vi "Parcial_Elevador.vi"() -> ()   [LabVIEW 2024]
uses:
  <vilib>/Utility/miscctls.llb/LVPositionTypeDef.ctl
panel:
  out "Position 2":T1
  in  "Position":T1={"Left"=400, "Top"=470}
  in  "Stop Button":bool
  in  "2 Piso Button":bool
  in  "3 Piso Button":bool
  in  "1 Piso Button":bool
  out "Elevador":bool
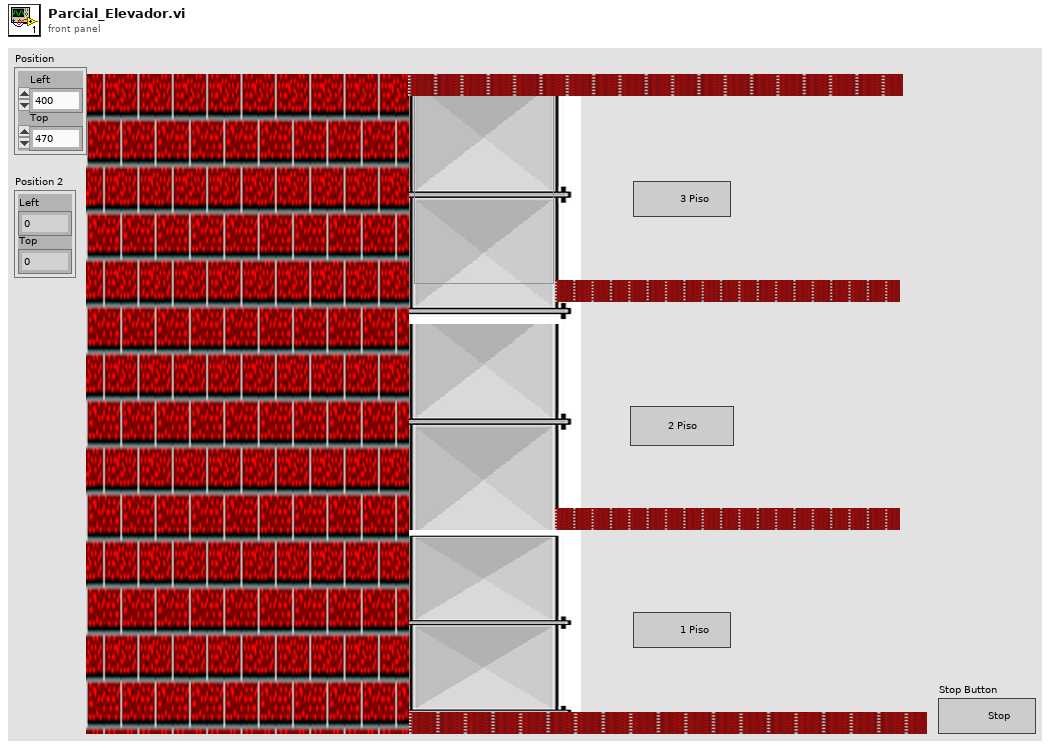
[diagram p1: front panel]
types:
  T1 = typedef "LVPositionTypeDef.ctl" = cluster{"Left":i32, "Top":i32}
  T2 = enum16{"Inicio", "1", "2 Subiendo", "3", "2 Bajando"}
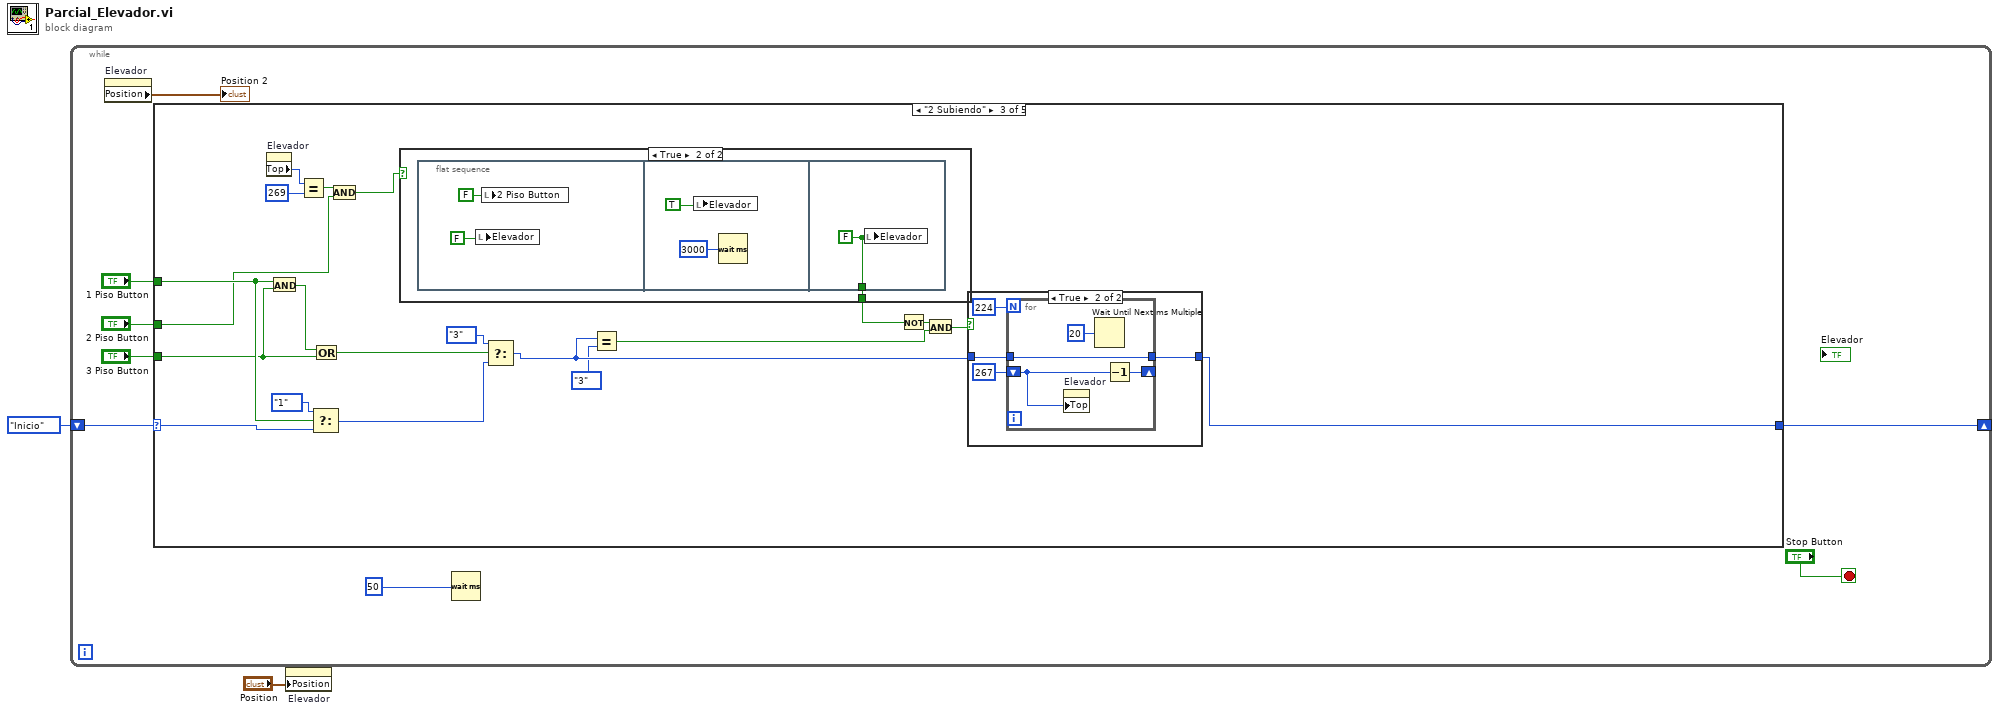
[diagram p0: block diagram]
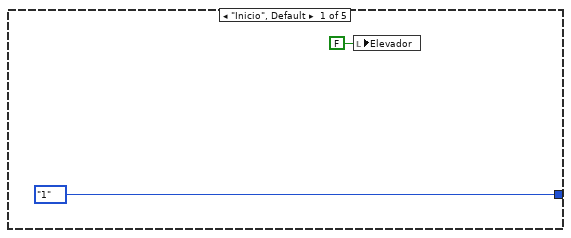
[diagram p2: hidden frame]
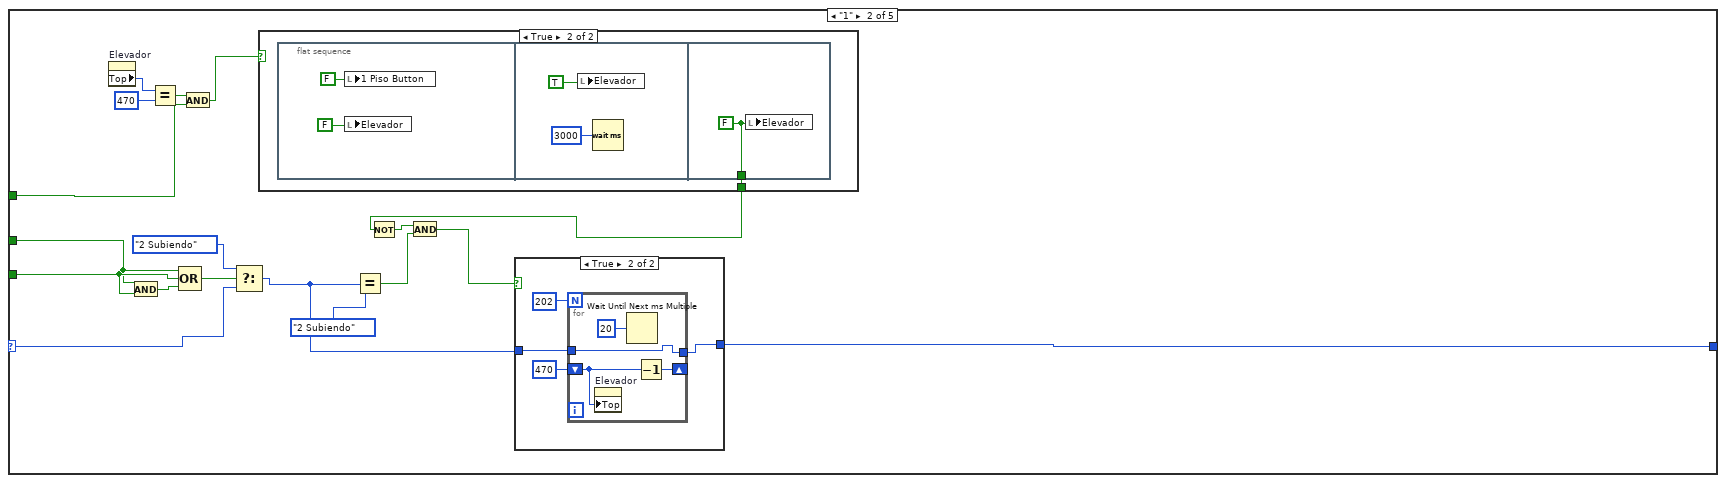
[diagram p3: hidden frame]
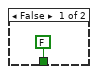
[diagram p5: hidden frame]
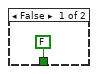
[diagram p6: hidden frame]
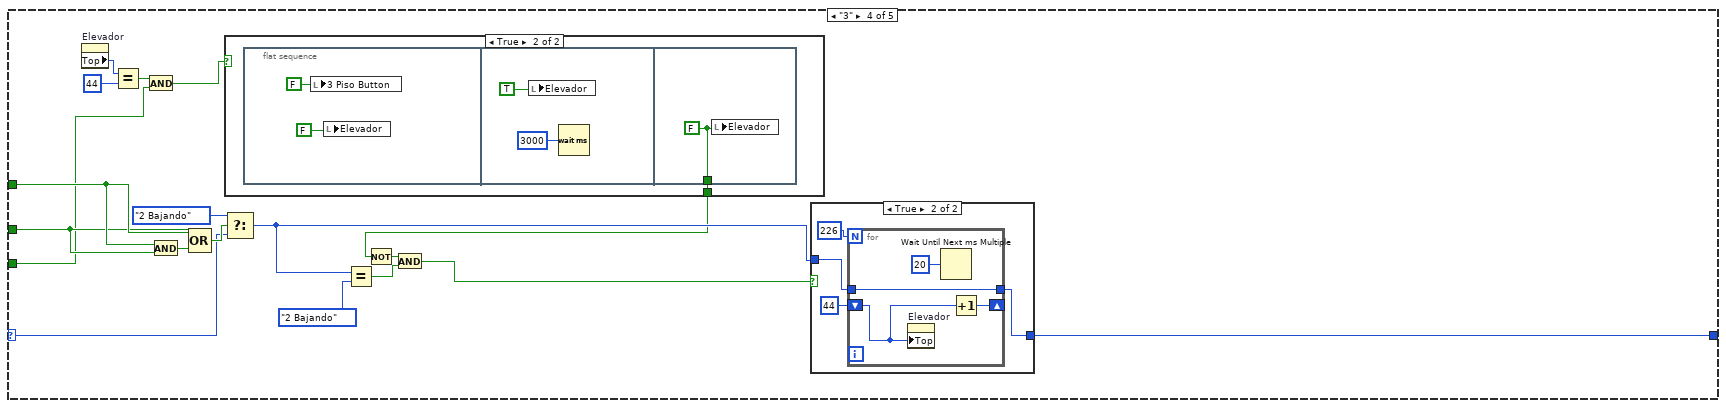
[diagram p8: hidden frame]
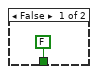
[diagram p9: hidden frame]
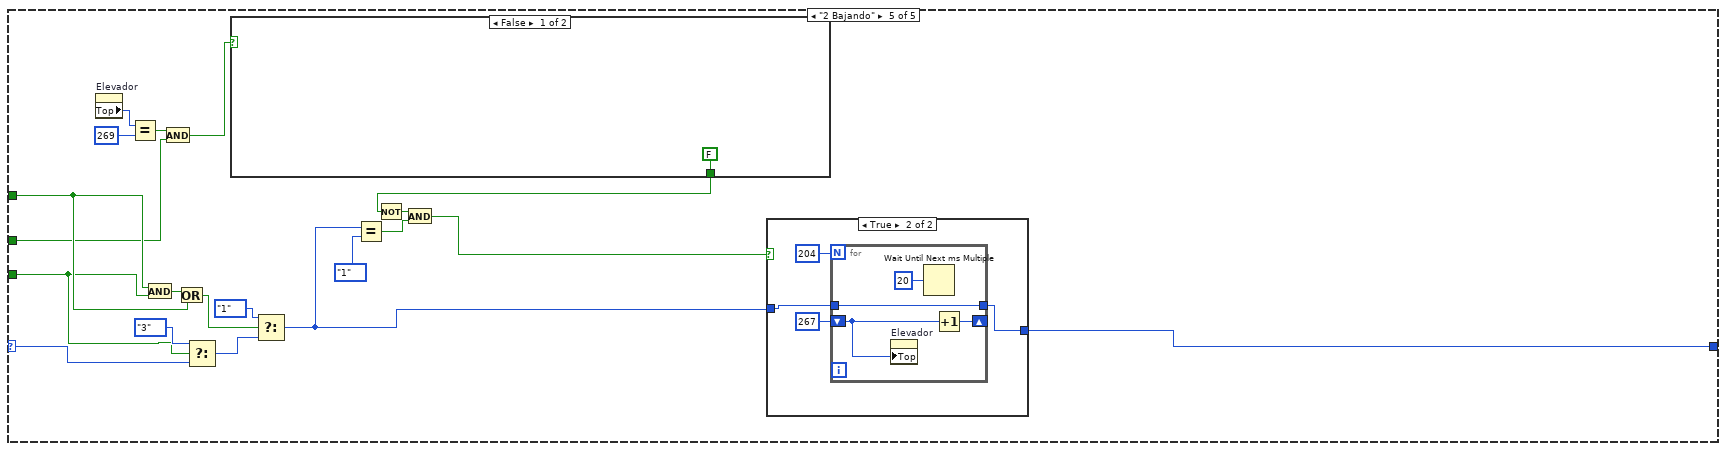
[diagram p11: hidden frame]
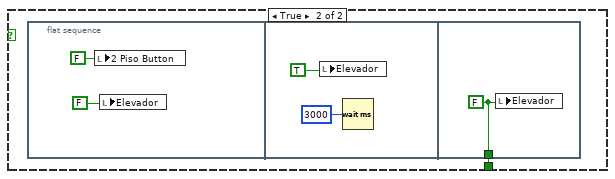
[diagram p12: hidden frame]
diagram:
  n1 = while {
    shift-right: [w4] -> _
    shift-left: T2."Inicio" -> [w9]
    stop <- "Stop Button" stop-if-true
    n2 = property on="Elevador" class="Bool (strict)"() -> ("Position"=→"Position 2":T1)  [unwired: 2 in, 2 out]
    n3 = case shown="\"2 Subiendo\"" w9 {
      selector: w9 -> [_ w25 w66 w92 w124]
      tunnel: [T2."1" w21 w59 w85 w125] -> w4
      tunnel: "1 Piso Button" -> [_ w16 w64 w99 w134]
      tunnel: "2 Piso Button" -> [_ w27 w49 w98 w126]
      tunnel: "3 Piso Button" -> [_ w28 w62 w91 w130]
      frame "Inicio", Default {
        n4 = local write "Elevador"(FALSE ("Elevador")) -> ()
      }
      frame "1" {
        n5 = property on="Elevador" class="Bool (strict)"() -> ("Top"=w19:i32)  [unwired: 2 in, 2 out]
        n6 = And(x=w27, y=w28) -> (x .and. y?=w29:bool)
        n7 = Equal?(x=w19, y=470) -> (x = y?=w17:bool)
        n8 = Compound Arithmetic op=OR(w27, w28, w29) -> (w26:bool)
        n9 = And(x=w17, y=w16) -> (x .and. y?=w15:bool)
        n10 = Select(t=T2."2 Subiendo", s=w26, f=w25) -> (s? t:f=w20:T2)
        n11 = case shown="True" w15 {
          tunnel: [FALSE w41] -> w13
          frame False {
          }
          frame True {
            n12 = flat-sequence {
              tunnel: [w46] -> w41
              frame #0 {
                n13 = local write "1 Piso Button"(FALSE ("1 Piso Button")) -> ()
                n14 = local write "Elevador"(FALSE) -> ()
              }
              frame #1 {
                n15 = local write "Elevador"(TRUE) -> ()
                n16 = Wait (ms)(milliseconds to wait=u32 3000) -> ()  [unwired: 1 out]
              }
              frame #2 {
                w46 = FALSE
                n17 = local write "Elevador"(w46) -> ()
              }
            }
          }
        }
        n18 = Equal?(x=w20, y=T2."2 Subiendo") -> (x = y?=w23:bool)
        n19 = Not(x=w13) -> (.not. x?=w14:bool)
        n20 = And(x=w14, y=w23) -> (x .and. y?=w22:bool)
        n21 = case shown="True" w22 {
          tunnel: [w31 w33] -> w21
          tunnel: w20 -> [w31 w32]
          frame False {
          }
          frame True {
            n22 = for {
              N: 202 -> [_]
              shift-right: [w38] -> _
              shift-left: 470 -> [w37]
              tunnel: [w36] -> w33
              tunnel: w32 -> [w36]
              n23 = property on="Elevador" class="Bool (strict)"("Top"=w37) -> ()  [unwired: 2 in, 2 out]
              n24 = Wait Until Next ms Multiple(millisecond multiple=u32 20 ("milliseconds to wait")) -> ()  [unwired: 1 out]
              n25 = Decrement(x=w37) -> (x-1=w38:i32)
            }
          }
        }
      }
      frame "2 Subiendo" {
        n26 = property on="Elevador" class="Bool (strict)"() -> ("Top"=w50:i32)  [unwired: 2 in, 2 out]
        n27 = And(x=w64, y=w62) -> (x .and. y?=w63:bool)
        n28 = Equal?(x=w50, y=269) -> (x = y?=w51:bool)
        n29 = Select(t=T2."1", s=w64, f=w66) -> (s? t:f=w57:T2)
        n30 = Or(x=w63, y=w62) -> (x .or. y?=w60:bool)
        n31 = And(x=w51, y=w49) -> (x .and. y?=w48:bool)
        n32 = case shown="True" w48 {
          tunnel: [FALSE w68] -> w47
          frame False {
          }
          frame True {
            n33 = flat-sequence {
              tunnel: [w73] -> w68
              frame #0 {
                n34 = local write "Elevador"(FALSE) -> ()
                n35 = local write "2 Piso Button"(FALSE ("1 Piso Button")) -> ()
              }
              frame #1 {
                n36 = local write "Elevador"(TRUE) -> ()
                n37 = Wait (ms)(milliseconds to wait=u32 3000) -> ()  [unwired: 1 out]
              }
              frame #2 {
                w73 = FALSE
                n38 = local write "Elevador"(w73) -> ()
              }
            }
          }
        }
        n39 = Select(t=T2."3", s=w60, f=w57) -> (s? t:f=w54:T2)
        n40 = Equal?(x=w54, y=T2."3") -> (x = y?=w55:bool)
        n41 = Not(x=w47) -> (.not. x?=w58:bool)
        n42 = And(x=w58, y=w55) -> (x .and. y?=w56:bool)
        n43 = case shown="True" w56 {
          tunnel: [w74 w76] -> w59
          tunnel: w54 -> [w74 w75]
          frame False {
          }
          frame True {
            n44 = for {
              N: 224 -> [_]
              shift-right: [w81] -> _
              shift-left: 267 -> [w80]
              tunnel: [w79] -> w76
              tunnel: w75 -> [w79]
              n45 = property on="Elevador" class="Bool (strict)"("Top"=w80) -> ()  [unwired: 2 in, 2 out]
              n46 = Wait Until Next ms Multiple(millisecond multiple=u32 20 ("milliseconds to wait")) -> ()  [unwired: 1 out]
              n47 = Decrement(x=w80) -> (x-1=w81:i32)
            }
          }
        }
      }
      frame "3" {
        n48 = property on="Elevador" class="Bool (strict)"() -> ("Top"=w93:i32)  [unwired: 2 in, 2 out]
        n49 = Equal?(x=w93, y=44) -> (x = y?=w94:bool)
        n50 = And(x=w94, y=w91) -> (x .and. y?=w84:bool)
        n51 = And(x=w99, y=w98) -> (x .and. y?=w100:bool)
        n52 = Compound Arithmetic op=OR(w99, w98, w100) -> (w97:bool)
        n53 = case shown="True" w84 {
          tunnel: [FALSE w102] -> w83
          frame False {
          }
          frame True {
            n54 = flat-sequence {
              tunnel: [w107] -> w102
              frame #0 {
                n55 = local write "3 Piso Button"(FALSE ("1 Piso Button")) -> ()
                n56 = local write "Elevador"(FALSE) -> ()
              }
              frame #1 {
                n57 = local write "Elevador"(TRUE) -> ()
                n58 = Wait (ms)(milliseconds to wait=u32 3000) -> ()  [unwired: 1 out]
              }
              frame #2 {
                w107 = FALSE
                n59 = local write "Elevador"(w107) -> ()
              }
            }
          }
        }
        n60 = Select(t=T2."2 Bajando", s=w97, f=w92) -> (s? t:f=w86:T2)
        n61 = Equal?(x=w86, y=T2."2 Bajando") -> (x = y?=w89:bool)
        n62 = Not(x=w83) -> (.not. x?=w90:bool)
        n63 = And(x=w90, y=w89) -> (x .and. y?=w87:bool)
        n64 = case shown="True" w87 {
          tunnel: w86 -> [w108 w112]
          tunnel: [w108 w111] -> w85
          frame False {
          }
          frame True {
            n65 = for {
              N: 226 -> [_]
              shift-right: [w113] -> _
              shift-left: 44 -> [w114]
              tunnel: [w115] -> w111
              tunnel: w112 -> [w115]
              n66 = property on="Elevador" class="Bool (strict)"("Top"=w114) -> ()  [unwired: 2 in, 2 out]
              n67 = Wait Until Next ms Multiple(millisecond multiple=u32 20 ("milliseconds to wait")) -> ()  [unwired: 1 out]
              n68 = Increment(x=w114) -> (x+1=w113:i32)
            }
          }
        }
      }
      frame "2 Bajando" {
        n69 = property on="Elevador" class="Bool (strict)"() -> ("Top"=w127:i32)  [unwired: 2 in, 2 out]
        n70 = Equal?(x=w127, y=269) -> (x = y?=w128:bool)
        n71 = And(x=w134, y=w130) -> (x .and. y?=w135:bool)
        n72 = And(x=w128, y=w126) -> (x .and. y?=w118:bool)
        n73 = Or(x=w135, y=w134) -> (x .or. y?=w133:bool)
        n74 = Select(t=T2."3", s=w130, f=w124) -> (s? t:f=w132:T2)
        n75 = case shown="False" w118 {
          tunnel: [FALSE w138] -> w117
          frame False {
          }
          frame True {
            n76 = flat-sequence {
              tunnel: [w143] -> w138
              frame #0 {
                n77 = local write "2 Piso Button"(FALSE ("1 Piso Button")) -> ()
                n78 = local write "Elevador"(FALSE) -> ()
              }
              frame #1 {
                n79 = local write "Elevador"(TRUE) -> ()
                n80 = Wait (ms)(milliseconds to wait=u32 3000) -> ()  [unwired: 1 out]
              }
              frame #2 {
                w143 = FALSE
                n81 = local write "Elevador"(w143) -> ()
              }
            }
          }
        }
        n82 = Select(t=T2."1", s=w133, f=w132) -> (s? t:f=w119:T2)
        n83 = Equal?(x=w119, y=T2."1") -> (x = y?=w122:bool)
        n84 = Not(x=w117) -> (.not. x?=w123:bool)
        n85 = And(x=w123, y=w122) -> (x .and. y?=w120:bool)
        n86 = case shown="True" w120 {
          tunnel: w119 -> [w144 w146]
          tunnel: [w144 w145] -> w125
          frame False {
          }
          frame True {
            n87 = for {
              N: 204 -> [_]
              shift-right: [w151] -> _
              shift-left: 267 -> [w150]
              tunnel: [w149] -> w145
              tunnel: w146 -> [w149]
              n88 = property on="Elevador" class="Bool (strict)"("Top"=w150) -> ()  [unwired: 2 in, 2 out]
              n89 = Wait Until Next ms Multiple(millisecond multiple=u32 20 ("milliseconds to wait")) -> ()  [unwired: 1 out]
              n90 = Increment(x=w150) -> (x+1=w151:i32)
            }
          }
        }
      }
    }
    n91 = Wait (ms)(milliseconds to wait=u32 50) -> ()  [unwired: 1 out]
  }
  n92 = property on="Elevador" class="Bool (strict)"("Position"="Position") -> ()  [unwired: 2 in, 2 out]
